vi "ProcessSpeedProfiles.vi"(8 "error in (no error)":errorcluster, 11 "tdms ref in":refnum<k34>) -> (0 "error out":errorcluster, 3 "tdms ref out":refnum<k34>)   [LabVIEW 2017, in "DataExplorerSupport.lvlib"]
uses:
  <vilib>/addons/InsightCM/Utilities/DataExplorerSupport/DataExplorerSupport.lvlib
  <vilib>/addons/InsightCM/Utilities/Tdms/Tdms.lvlib
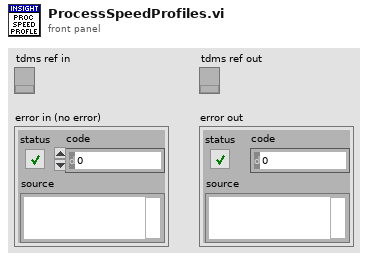
[diagram p1: front panel]
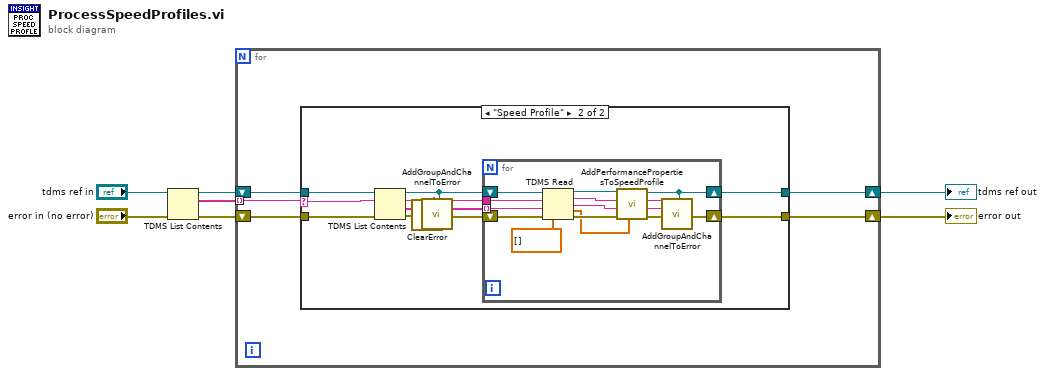
[diagram p0: block diagram]
diagram:
  n1 = TDMS List Contents(4:"error in (no error)", 7:"tdms ref in") -> (0:w4:errorcluster, 2:w1:string[], 3:w3:refnum<k34>)  [unwired: 1 in, 1 out]
  n2 = for {
    shift-right: [w12] -> w7
    shift-left: w4 -> [w10]
    shift-right: [w11] -> w6
    shift-left: w3 -> [w9]
    tunnel: w1 -> [w8] mode=indexing
    n3 = case shown="\"Speed Profile\"" w8 {
      selector: w8 -> [_ w15]
      tunnel: [w13 w21] -> w12
      tunnel: [w14 w20] -> w11
      tunnel: w10 -> [w13 w17]
      tunnel: w9 -> [w14 w16]
      frame Default {
      }
      frame "Speed Profile" {
        n4 = TDMS List Contents(4:w17, 6:w15, 7:w16) -> (0:w18:errorcluster, 1:w19:string[], 2:w22:string, 3:w23:refnum<k34>)
        n5 = call <vilib>:"ClearError.vi"("error in (no error)"=w18) -> ("error out"=w25:errorcluster)
        n6 = call <vilib>:"AddGroupAndChannelToError.vi"("error in (no error)"=w25, "group name in"=w22, "Refnum in"=w23) -> ("error out"=w24:errorcluster)  [unwired: 16 in]
        n7 = for {
          tunnel: w19 -> [w38] mode=indexing
          tunnel: w22 -> [w39]
          shift-right: [w35] -> w21
          shift-left: w24 -> [w37]
          shift-right: [w29] -> w20
          shift-left: w23 -> [w40]
          n8 = TDMS Read(0:w40, 5:w39, 7:w38, 11:w37, 12:dbl[] [] ("Array")) -> (4:w30:refnum<k34>, 6:w31:string, 8:w32:string, 10:w33:dbl[], 15:w34:errorcluster)  [unwired: 3 in, 1 out]
          n9 = call <vilib>:"AddPerformancePropertiesToSpeedProfile.vi"("Speed Profile"=w33, "error in (no error)"=w34, "Channel"=w32, "Group"=w31, "Tdms Ref"=w30) -> ("error out"=w26:errorcluster, "Channel out"=w27:string, "Group out"=w28:string, "Tdms Ref out"=w29:refnum<k34>)  [unwired: 3 in]
          n10 = call <vilib>:"AddGroupAndChannelToError.vi"("error in (no error)"=w26, "channel name in"=w27, "group name in"=w28, "Refnum in"=w29) -> ("error out"=w35:errorcluster)  [unwired: 15 in]
        }
      }
    }
  }
  "error out" <- w7
  "tdms ref out" <- w6
